vi "MacroBasher.vi"(4 "Changes":bool[][](array[boolean]), 5 "Path tag":string, 6 "Total time (s)":dbl, 7 "Instructions":T1 {"Steps" min=1 max=100000 step=1; "Duration" min=0.001 step=0.001 format="%_6p"}, 9 "Macro Description":string, 10 "Variable Cluster":T3 {"Variable Type" items=["Duration (s)", "Voltage (V)", "Parameter"]; "Final Val" format="%_6p"; "First Val" format="%_6p"; "Values" format="%_6p"}, 11 "Save/Open Path":path) -> ()   [LabVIEW 2018]
uses:
  Executor Files/VariableScan_Cluster.ctl
  Instructions.ctl
  Executor Files/RT/Instruction.ctl
  MacroSaveCluster.ctl
  <vilib>/Analysis/1siggen.llb/Ramp Pattern by Samples.vi
  <vilib>/Analysis/NI_AALBase.lvlib
panel:
  # "0        2       4       6        8      10     12     14     16     18      20    22     24     26     28     30     32     34     36"
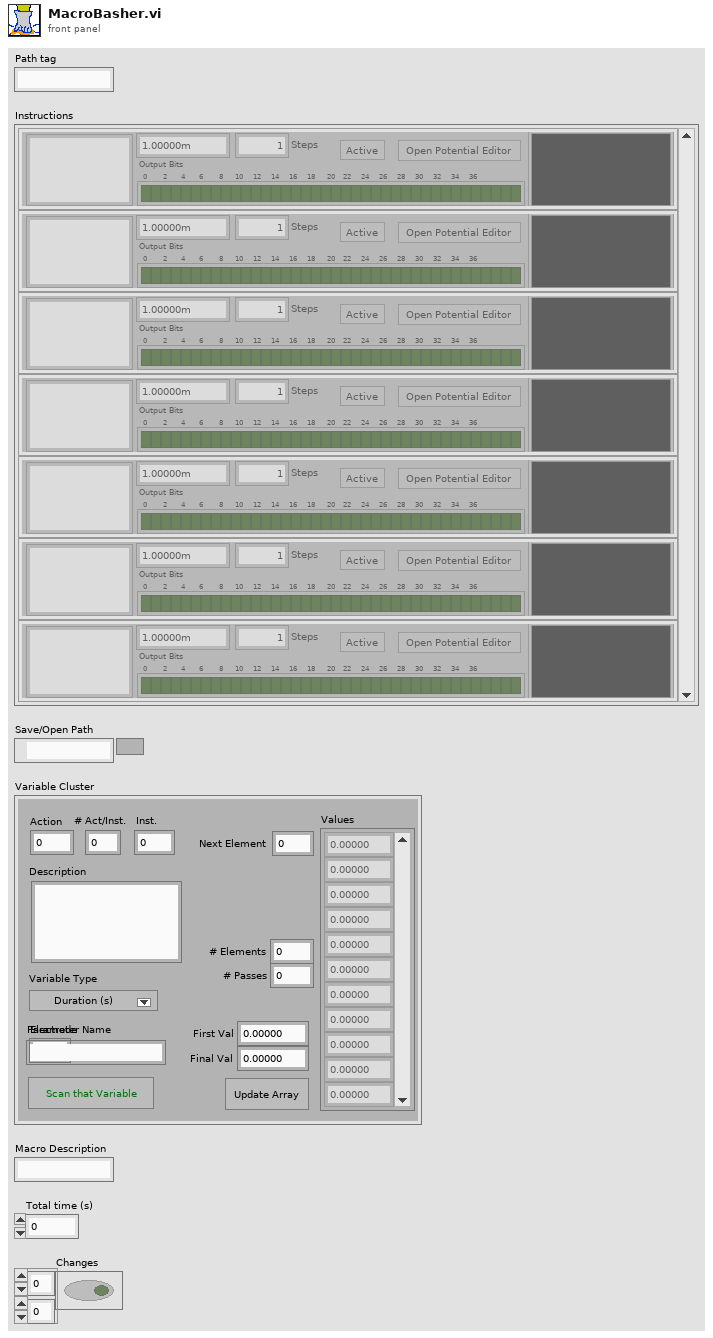
[diagram p1: front panel]
types:
  T1 = typedef "Instructions.ctl" = T2[]
  T2 = typedef "Instruction.ctl" = cluster{"Duration":dbl, "Comment":string, "Steps":i32, "Edit Potential":bool, "Output Bits":bool[], "Macro Path":path, "Potentials":dbl[], "Inherit?":bool}
  T3 = typedef "VariableScan_Cluster.ctl" = cluster{"Values":dbl[], "Action":i32, "Inst.":i32, "# Elements":i32, "Next Element":i32, "First Val":dbl, "Final Val":dbl, "Update Array":bool, "Description":string, "Variable Type":u16, "Scan Now":bool, "# Act/Inst.":i32, "Electrode":i32, "Parameter Name":string, "# Passes":i32}
  T4 = typedef "MacroSaveCluster.ctl" = cluster{"Instructions":T1, "Changes":bool[][], "Macro Description":string, "Total Time (s)":dbl, "Samples per sec":dbl}
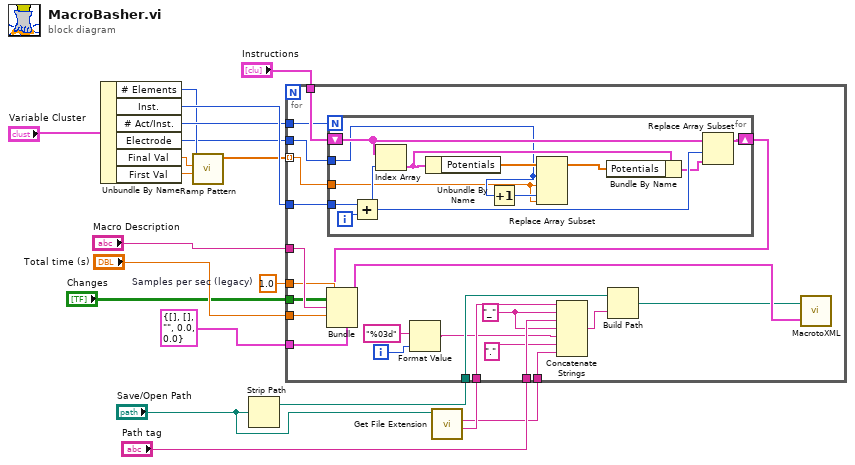
[diagram p0: block diagram]
diagram:
  w10 = 1.0  # Samples per sec (legacy)
  n1 = Unbundle By Name("Variable Cluster") -> ("# Elements"=w13:i32, "Inst."=w16:i32, "# Act/Inst."=w15:i32, "Electrode"=w3:i32, "Final Val"=w11:dbl, "First Val"=w12:dbl)
  n2 = call-poly <vilib>:"Ramp Pattern.vi"("start"=w12, "end"=w11, "samples"=w13) -> ("Ramp Pattern"=w14:dbl[])  [unwired: 7 in, 1 out]
  n3 = Strip Path(path="Save/Open Path") -> (stripped path=w17:path)  [unwired: 1 out]
  n4 = call <vilib>:"Get File Extension.vi"("file"="Save/Open Path") -> ("filename without extension"=w18:string, "lowercase file extension"=w2:string)  [unwired: 6 in, 3 out]
  n5 = for {
    tunnel: "Instructions" -> [w35]
    tunnel: "Macro Description" -> [w42]
    tunnel: "Changes" -> [w41]
    tunnel: "Total time (s)" -> [w39]
    tunnel: T4 {"Instructions"=[], "Changes"=[], "Macro Description"="", "Total Time (s)"=0.0, "Samples per sec"=0.0} ("output cluster") -> [w38]
    tunnel: w10 -> [w37]
    tunnel: w14 -> [w31] mode=indexing
    tunnel: w15 -> [w34]
    tunnel: w16 -> [w33]
    tunnel: w17 -> [w30]
    tunnel: w18 -> [w29]
    tunnel: "Path tag" -> [w28]
    tunnel: w3 -> [w32]
    tunnel: w2 -> [w23]
    i -> [w22]
    w27 = "_" ("string")
    n6 = for {
      N: w34 -> [_]
      shift-right: [w54] -> w36
      shift-left: w35 -> [w53]
      tunnel: w33 -> [w51]
      tunnel: w32 -> [w44]
      tunnel: w31 -> [w43]
      i -> [w52]
      n7 = Add(x=w51, y=w52) -> (x+y=w50:i32)
      n8 = Index Array(array=w53, index=w50) -> (element=w47:T2)
      n9 = Unbundle By Name(w47) -> ("Potentials"=w49:dbl[])
      n10 = Increment(x=w44) -> (x+1=w45:i32)
      n11 = Replace Array Subset(array=w49, new element #1=w43, index #1=w44, new element #2=w43, index #2=w45) -> (w48:dbl[])
      n12 = Bundle By Name(cluster=w47, "Potentials"=w48) -> (w46:T2)
      n13 = Replace Array Subset(array=w53, new element=w46, index=w50) -> (w54:T1)
    }
    n14 = Bundle(cluster=w38, "Instructions"=w36, "Changes"=w41, "Macro Description"=w42, "Total Time (s)"=w39, "Samples per sec"=w37) -> (w40:T4)
    n15 = Format Value(format string="%03d", value (0)=w22) -> (output string=w21:string)  [unwired: 1 in]
    n16 = Concatenate Strings(w29, w27, w28, w27, w21, "." ("string"), w23) -> (w26:string)
    n17 = Build Path(base path=w30, name or relative path=w26) -> (appended path=w25:path)
    n18 = call "MacrotoXML.vi"("MacroSaveCluster"=w40, "XML File Path"=w25) -> ()  [unwired: 1 in]
  }
